vi "Memory Usage Monitoring.vi"() -> ()   [LabVIEW 2016]
doc: "The Task Monitor uses .NET assemblies to monitor basic CPU and system memory usage. It uses the PerformanceCounter class to get the CPU usage and also to determine how much memory is being used. \n\nThe example makes use of the System.Diagnostics.PerformanceCounter class. The PerformanceCounter category names and counterNames were obtained from the Microsoft documentation for the PerformanceCounter class. For more information about the various .NET libraries used in this example, refer to the Microsoft Developers Network at msdn.microsoft.com."
uses:
  Core/Assert API Components/Assert API Components.lvlib
panel:
  out "Data":T1(graph)
  out "Number of Asserts":i32
  in  "Stop":bool
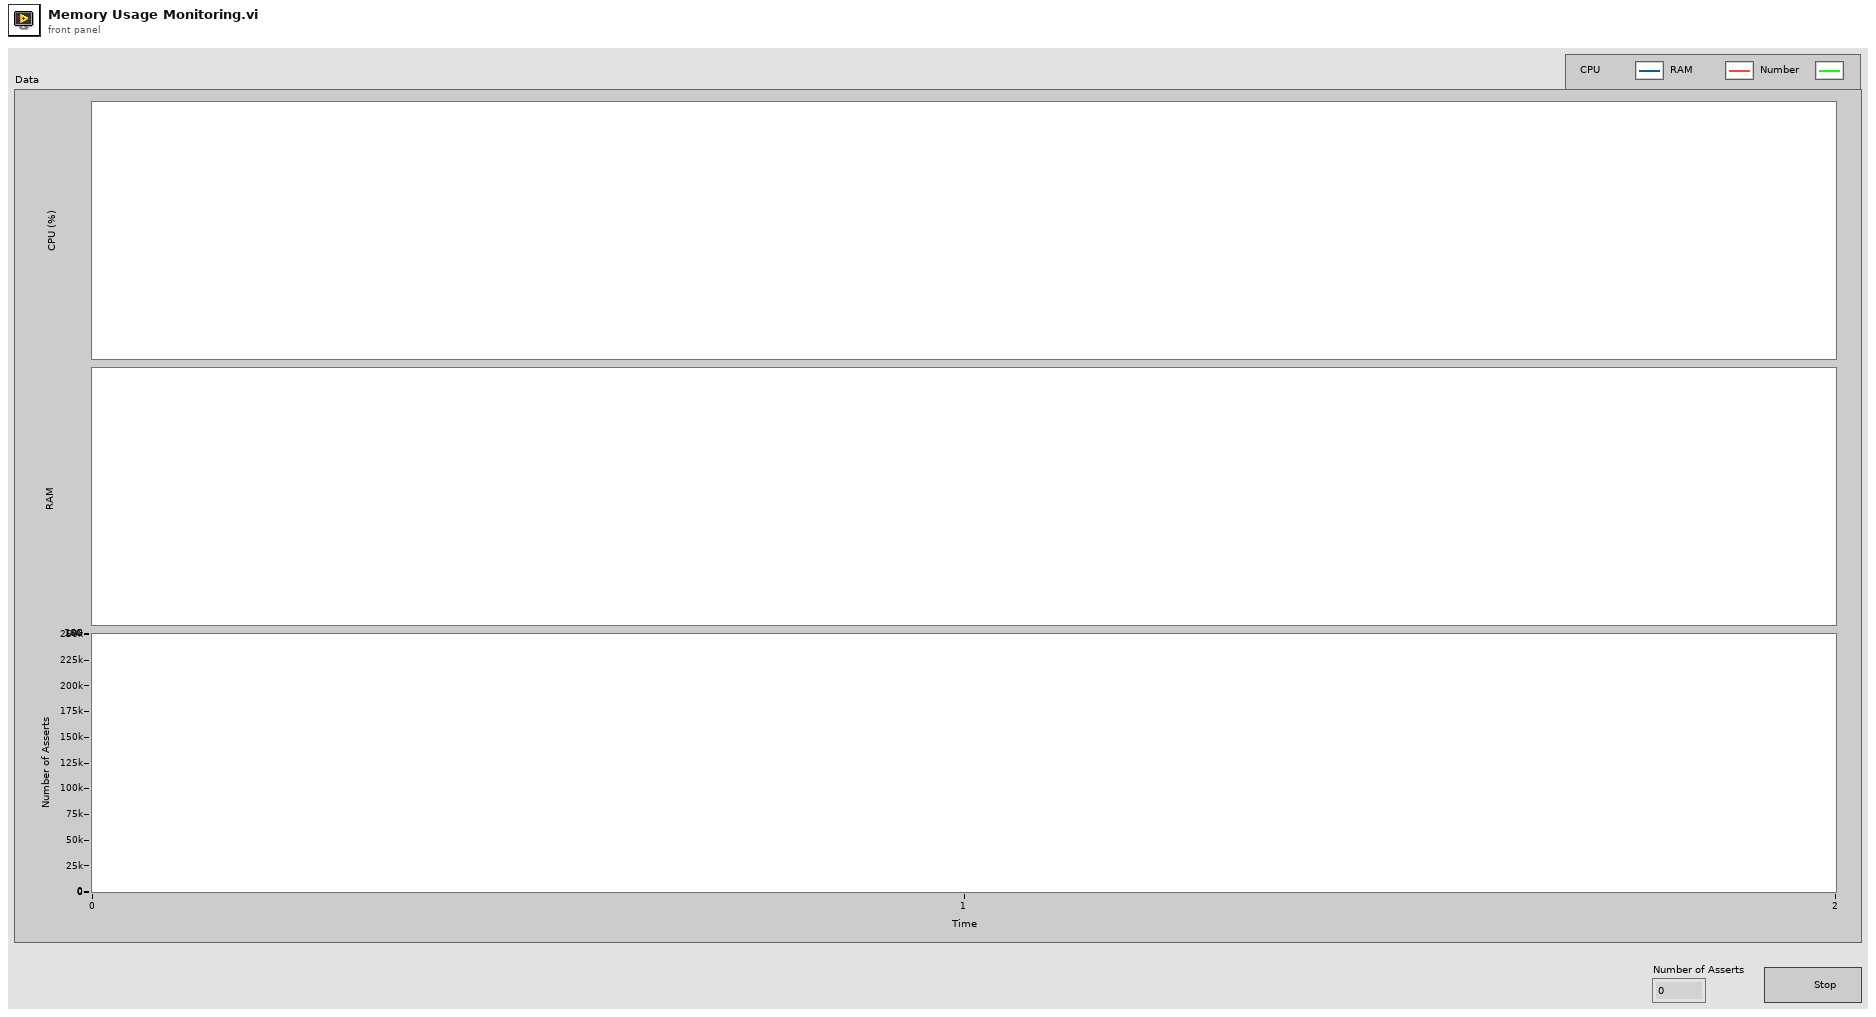
[diagram p1: front panel]
types:
  T1 = cluster{"NextValue":sgl, "NextValue":sgl, "Number of Asserts":i32}
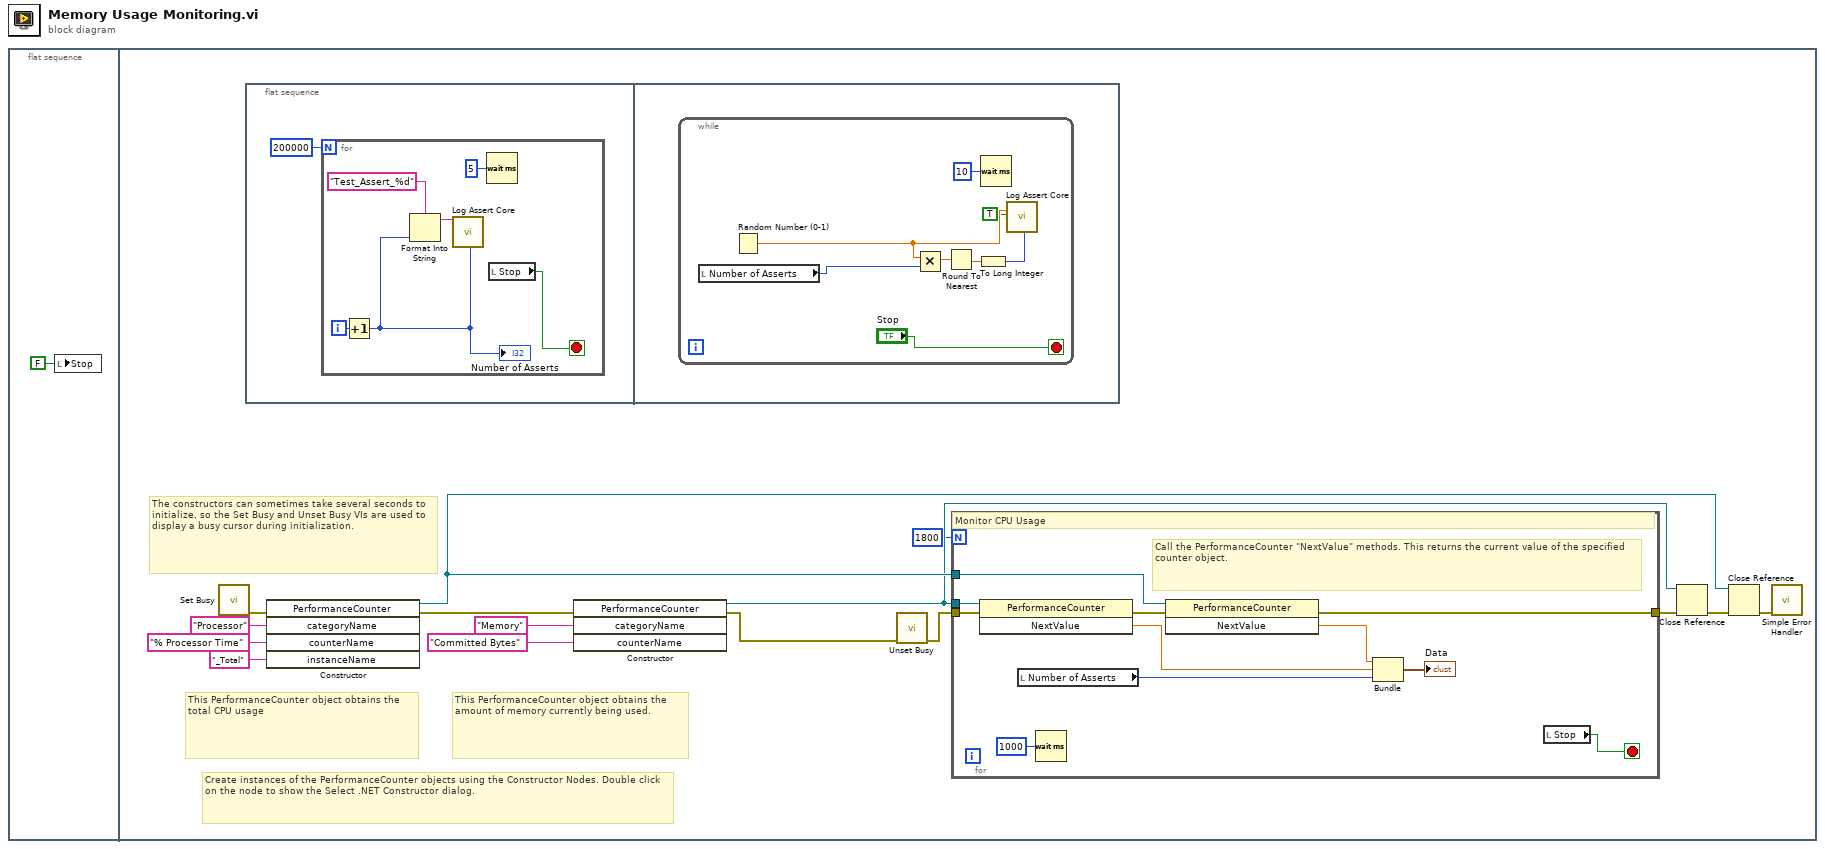
[diagram p0: block diagram]
diagram:
  n1 = flat-sequence {
    frame #0 {
      n2 = local write "Stop"(FALSE ("Stop")) -> ()
    }
    frame #1 {
      # "The constructors can sometimes take several seconds to initialize, so the Set Busy and Unset Busy VIs are used to display a busy cursor during initialization."
      # "Create instances of the PerformanceCounter objects using the Constructor Nodes. Double click on the node to show the Select .NET Constructor dialog."
      # "This PerformanceCounter object obtains the amount of memory currently being used."
      # "This PerformanceCounter object obtains the total CPU usage"
      n3 = call <vilib>:"Set Busy.vi"() -> ("error out"=w5:errorcluster)  [unwired: 10 in, 1 out]
      n4 = flat-sequence {
        frame #0 {
          n5 = for {
            N: 200000 -> [_]
            i -> [w34]
            stop <- w29 stop-if-true
            n6 = Increment(x=w34) -> (x+1=w30:i32)
            "Number of Asserts" <- w30
            n7 = Format Into String(format string="Test_Assert_%d", w30) -> (resulting string=w33:string)  [unwired: 2 in, 1 out]
            n8 = call "Log Assert Core.vi"("Assert Name"=w33, "Assert VI UID"=w30) -> ()  [unwired: 18 in]
            n9 = Wait (ms)(milliseconds to wait=u32 5) -> ()  [unwired: 1 out]
            n10 = local read "Stop"() -> (w29:bool)
          }
        }
        frame #1 {
          n11 = while {
            stop <- "Stop" stop-if-true
            n12 = local read "Number of Asserts"() -> (w42:i32)
            n13 = Random Number (0-1)() -> (number: 0 to 1=w36:dbl)
            n14 = Multiply(x=w36, y=w42) -> (x*y=w41:dbl)
            n15 = Round To Nearest(number=w41) -> (nearest integer value=w40:dbl)
            n16 = To Long Integer(number=w40) -> (32bit integer=w39:i32)
            n17 = Wait (ms)(milliseconds to wait=u32 10) -> ()  [unwired: 1 out]
            n18 = call "Log Assert Core.vi"("Data Value"=w36, "Status"=TRUE, "Assert VI UID"=w39) -> ()  [unwired: 17 in]
          }
        }
      }
      n19 = constructor class="PerformanceCounter"(error in=w5, "categoryName"="Processor", "counterName"="% Processor Time", "instanceName"="_Total") -> (reference out=w7:refnum<k24>, error out=w12:errorcluster)  [unwired: 2 in, 4 out]
      n20 = constructor class="PerformanceCounter"(error in=w12, "categoryName"="Memory", "counterName"="Committed Bytes") -> (reference out=w6:refnum<k24>, error out=w4:errorcluster)  [unwired: 2 in, 3 out]
      n21 = call <vilib>:"Unset Busy.vi"("error in (no error)"=w4) -> ("error out"=w3:errorcluster)  [unwired: 10 in]
      n22 = for {
        N: 1800 -> [_]
        tunnel: w7 -> [w26]
        tunnel: w6 -> [w25]
        tunnel: w3 -> [w23]
        tunnel: [w24] -> w11
        stop <- w17 stop-if-true
        # "Call the PerformanceCounter \"NextValue\" methods. This returns the current value of the specified counter object."
        # "Monitor CPU Usage"
        n23 = invoke class="PerformanceCounter" method="NextValue"(reference=w25, error in=w23) -> (error out=w22:errorcluster, "NextValue"=w20:sgl)  [unwired: 1 in, 1 out]
        n24 = local read "Number of Asserts"() -> (w19:i32)
        n25 = Wait (ms)(milliseconds to wait=u32 1000 ("millisecond multiple")) -> ()  [unwired: 1 out]
        n26 = invoke class="PerformanceCounter" method="NextValue"(reference=w26, error in=w22) -> (error out=w24:errorcluster, "NextValue"=w21:sgl)  [unwired: 1 in, 1 out]
        n27 = Bundle("NextValue"=w21, "NextValue"=w20, "Number of Asserts"=w19) -> (→"Data":T1)  [unwired: 1 in]
        n28 = local read "Stop"() -> (w17:bool)
      }
      n29 = Close Reference(reference=w6, error in (no error)=w11) -> (error out=w13:errorcluster)
      n30 = Close Reference(reference=w7, error in (no error)=w13) -> (error out=w14:errorcluster)
      n31 = call <vilib>:"Simple Error Handler.vi"("error in (no error)"=w14) -> ()  [unwired: 1 in, 8 out]
    }
  }
